vi "FTW-Ether-Connections-AE.vi"(0 "Connection":string, 2 "Action":T1, 5 "Address":string, 11 "error in":errorcluster) -> (6 "Fetched Address":string, 15 "error out":errorcluster)   [LabVIEW 2015, in "FTW-Ether.lvclass"]
uses:
  FTW-Ether.lvclass
  FTW-Ether-Connections-Action.ctl
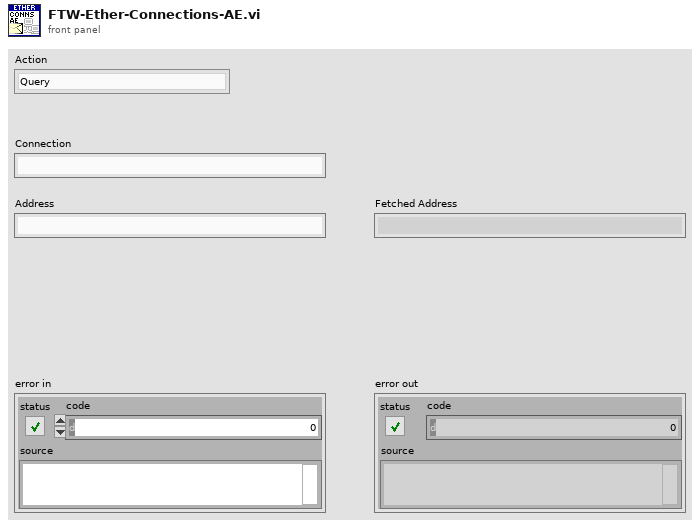
[diagram p1: front panel]
types:
  T1 = typedef "FTW-Ether.lvclass/FTW-Ether-Connections-Action.ctl" = enum8{"Query", "Add", "Reset"}
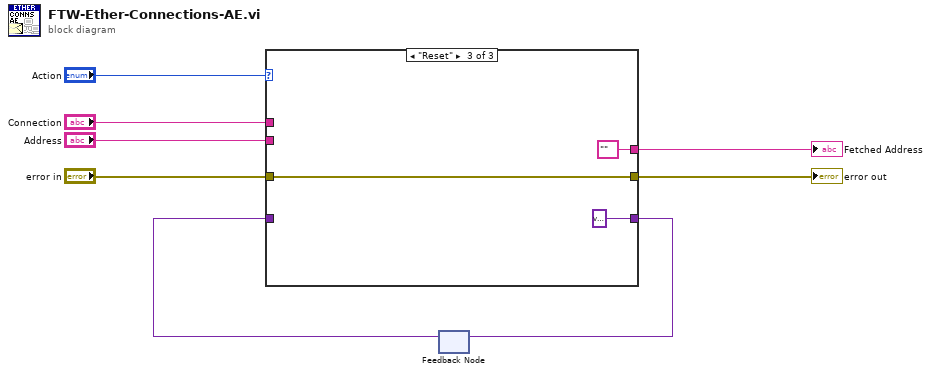
[diagram p0: block diagram]
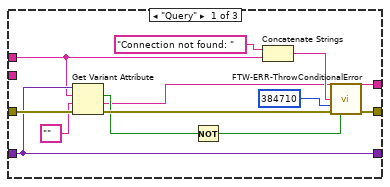
[diagram p2: hidden frame]
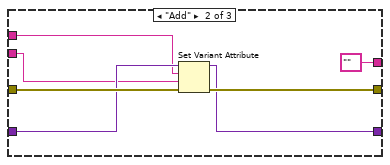
[diagram p3: hidden frame]
diagram:
  n1 = feedback #1() -> (w3:variant)  [unwired: 1 in]
  n2 = case shown="\"Reset\"" "Action" {
    tunnel: "Connection" -> [w12 w22 _]
    tunnel: [w9 "" ("empty string") "" ("empty string")] -> w6
    tunnel: "Address" -> [_ w21 _]
    tunnel: [w13 w23 variant] -> w4
    tunnel: w3 -> [w13 w24 _]
    tunnel: "error in" -> [w20 w26 w30]
    tunnel: [w19 w25 w30] -> w1
    frame "Query" {
      n3 = Get Variant Attribute(Variant=w13, name=w12, default value (empty Variant)="" ("empty string"), error in=w20) -> (found=w10:bool, value=w9:string, error out=w14:errorcluster)  [unwired: 1 out]
      n4 = Not(x=w10) -> (.not. x?=w18:bool)
      n5 = Concatenate Strings("Connection not found: " ("Error Message"), w12) -> (w15:string)
      n6 = call "FTW-ERR-ThrowConditionalError.vi"("Error Message"=w15, "Error Code"=384710, "error in"=w14, "Throw Error?"=w18) -> ("error out"=w19:errorcluster)  [unwired: 11 in]
    }
    frame "Add" {
      n7 = Set Variant Attribute(Variant=w24, name=w22, value=w21, error in=w26) -> (Variant out=w23:variant, error out=w25:errorcluster)  [unwired: 1 out]
    }
    frame "Reset" {
    }
  }
  "Fetched Address" <- w6
  "error out" <- w1
  n8 = feedback-in #1(w4) -> ()
